vi "array.vi"() -> ()   [LabVIEW 2021]
panel:
  out "Waveform Graph":cluster{i32, i32, dbl[]}(graph)
  out "1-array":dbl[](array[numeric])
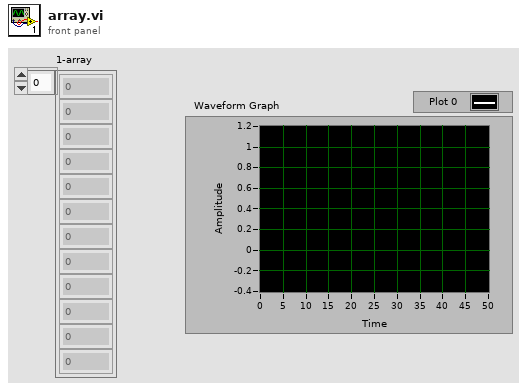
[diagram p1: front panel]
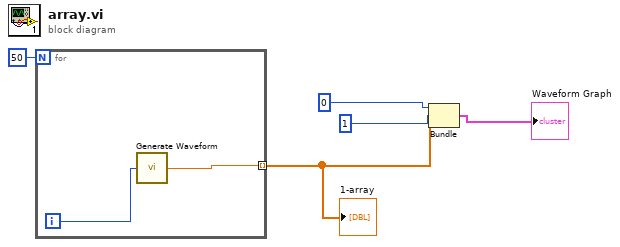
[diagram p0: block diagram]
diagram:
  n1 = for {
    N: 50 -> [_]
    tunnel: [w6] -> w5 mode=indexing
    i -> [w7]
    n2 = call "Generate Waveform.vi"("Index"=w7) -> ("Waveform Point"=w6:dbl)
  }
  "1-array" <- w5
  n3 = Bundle(0, 1, w5) -> (→"Waveform Graph":cluster{i32, i32, dbl[]})  [unwired: 1 in]
